vi "Host - Launch Target VIs (SubVI).vi"(8 "error in":errorcluster, 11 "IP":string[](array[string])) -> (0 "error out":errorcluster, 1 "VI Ref":refnum<vi>[](array[refnum]), 2 "Channel Data":cluster{"AI":T5, "DI":T2, "DO":T2, "Async":T9}[](array[cluster]) {"AI"."Interface Data"."Timing"."sample mode" items=["Finite Samples"=10178, "Continuous Samples"=10123, "Hardware Timed Single Point"=12522]; "Async"."Interface Data"."Data"."Minor Frame Count" min=5 max=8 step=1}, 3 "DO":T2[](array[typedef]), 7 "DI":T2[](array[typedef]))   [LabVIEW 2021]
uses:
  Async Serial/Controls/Async Message Info Cluster.ctl
  Async Serial/Controls/Async Frame Info Cluster.ctl
  Async Serial/Controls/Async Serial Configuration Cluster.ctl
  Async Interface Data Cluster.ctl
  Async JSON Cluster.ctl
  Digital Output/SubVIs/Digital Dynamic Cluster.ctl
  Digital Output/Controls/DIO Interface Data.ctl
  Digital Output/Controls/DIO Configuration cluster.ctl
  Analog Output/Controls/AO Timing Cluster.ctl
  Analog Output/Controls/AO Channel Configuration Cluster.ctl
  Analog Output/Controls/AO Interface Data Cluster.ctl
  Analog Output/Controls/AO JSON Data Cluster.ctl
  Async Serial/Controls/Async Sensor Type.ctl
panel:
  in  "Sensor Type":T1=enum."INS"
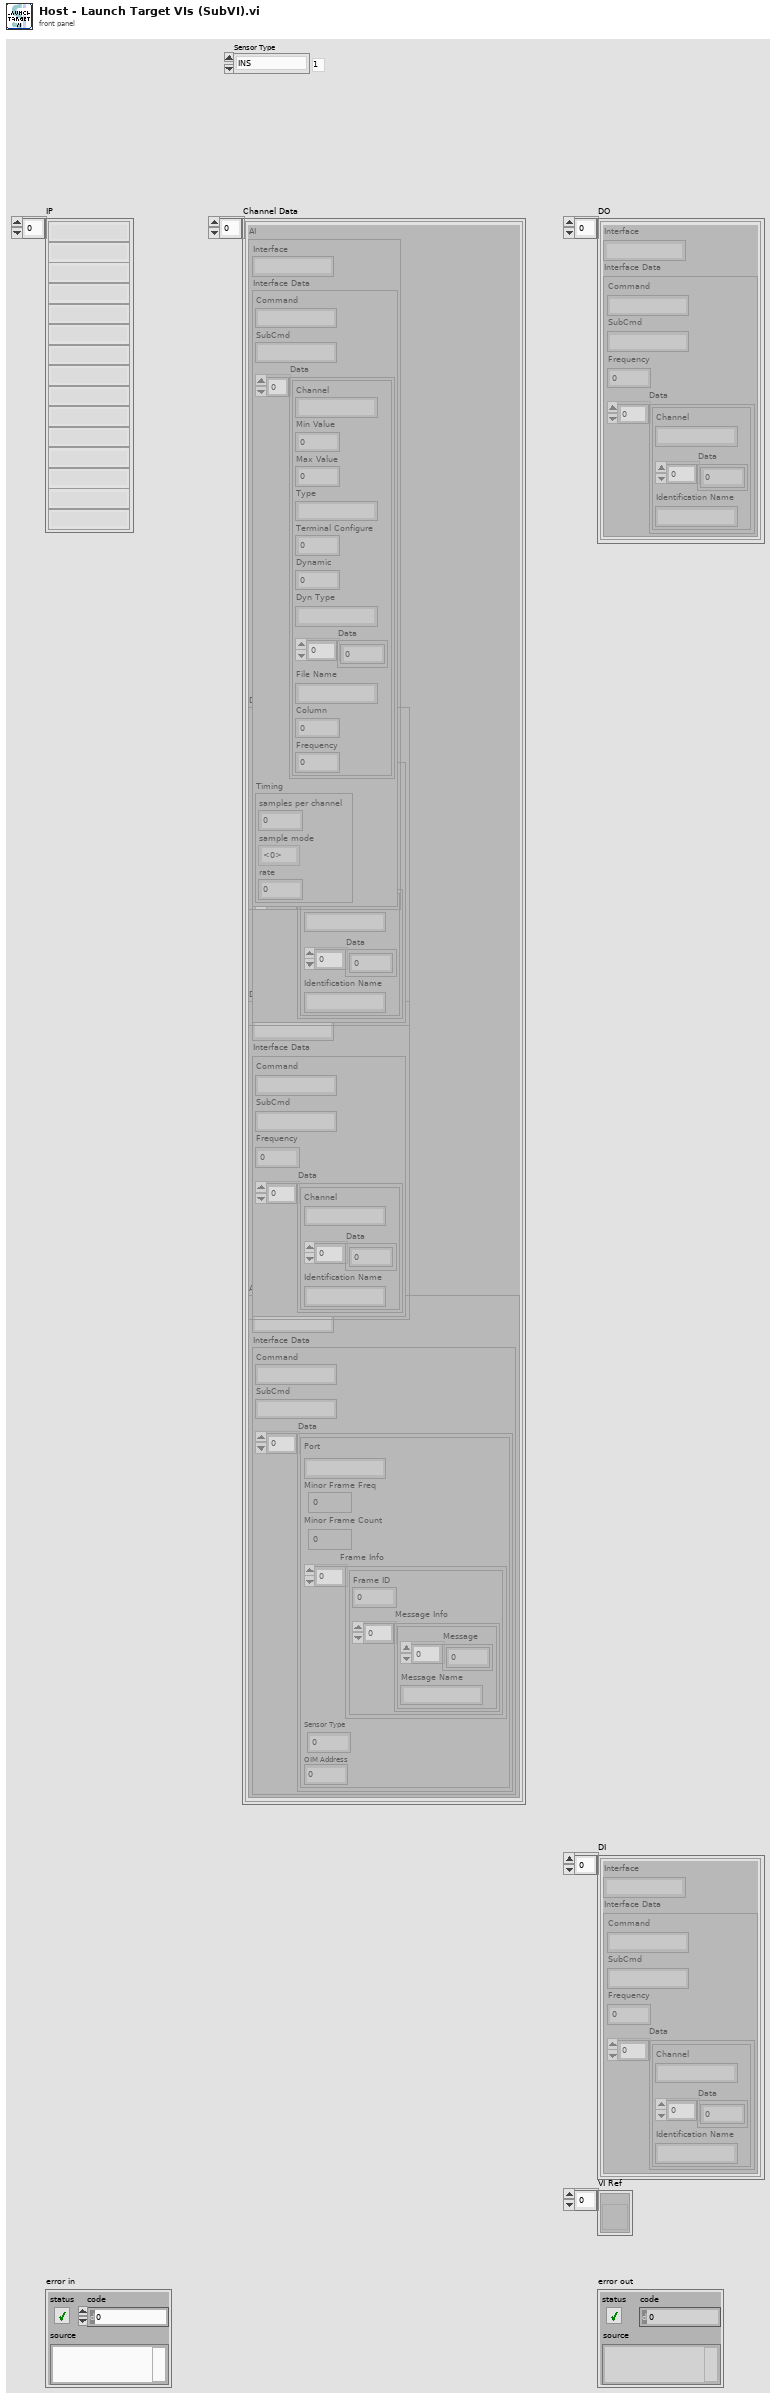
[diagram p1: front panel]
types:
  T1 = typedef "Async Sensor Type.ctl" = enum16{"Camera", "INS", "Pri BMS", "Aux BMS", "Depth Sensor", "Altimeter", "OIM", "Thruster", "Acoustic Modem", "LED"}
  T2 = typedef "DIO Configuration cluster.ctl" = cluster{"Interface":string, "Interface Data":T3}
  T3 = typedef "DIO Interface Data.ctl" = cluster{"Command":string, "SubCmd":string, "Frequency":u16, "Data":T4[]}
  T4 = typedef "Digital Dynamic Cluster.ctl" = cluster{"Channel":string, "Data":u8[], "Identification Name":string}
  T5 = typedef "AO JSON Data Cluster.ctl" = cluster{"Interface":string, "Interface Data":T6}
  T6 = typedef "AO Interface Data Cluster.ctl" = cluster{"Command":string, "SubCmd":string, "Data":T7[], "Timing":T8}
  T7 = typedef "AO Channel Configuration Cluster.ctl" = cluster{"Channel":string, "Min Value":dbl, "Max Value":dbl, "Type":string, "Terminal Configure":u16, "Dynamic":u8, "Dyn Type":string, "Data":dbl[], "File Name":string, "Column":i32, "Frequency":dbl}
  T8 = typedef "AO Timing Cluster.ctl" = cluster{"samples per channel":i32, "sample mode":i32, "rate":dbl}
  T9 = typedef "Async JSON Cluster.ctl" = cluster{"Interface":string, "Interface Data":T10}
  T10 = typedef "Async Interface Data Cluster.ctl" = cluster{"Command":string, "SubCmd":string, "Data":T11[]}
  T11 = typedef "Async Serial Configuration Cluster.ctl" = cluster{"Port":string, "Minor Frame Freq":u16, "Minor Frame Count":u16, "Frame Info":T12[], "Sensor Type":u16, "OIM Address":u16}
  T12 = typedef "Async Frame Info Cluster.ctl" = cluster{"Frame ID":u16, "Message Info":T13[]}
  T13 = typedef "Async Message Info Cluster.ctl" = cluster{"Message":u8[], "Message Name":string}
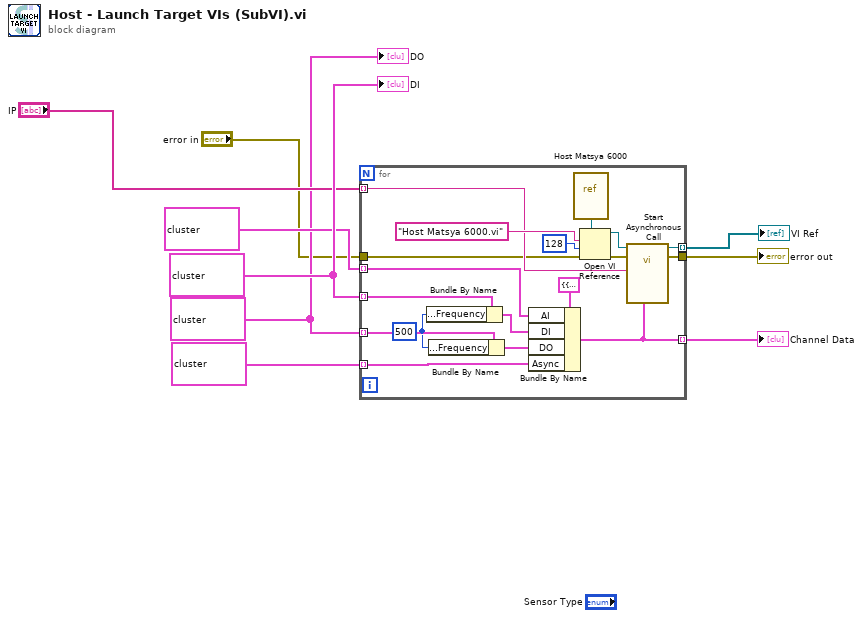
[diagram p0: block diagram]
diagram:
  w9 = T2[] [{"Interface"="DIO", "Interface Data"={"Command"="Configure", "SubCmd"="DI", "Frequency"=500, "Data"=[{"Channel"="Mod3/port0/line0", "Data"=[0], "Identification Name"=""}, {"Channel"="Mod3/port0/line1", "Data"=[0], "Identification Name"=""}, {"Channel"="Mod3/port0/line2", "Data"=[0], "Identification Name"=""}, {"Channel"="Mod3/port0/line3", "Data"=[0], "Identification Name"=""}, {"Channel"="Mod3/port0/line4", "Data"=[0], "Identification Name"=""}, {"Channel"="Mod3/port0/line5", "Data"=[0], "Identification Name"=""}, {"Channel"="Mod3/port0/line6", "Data"=[0], "Identification Name"=""}, {"Channel"="Mod3/port0/line7", "Data"=[0], "Identification Name"=""}, {"Channel"="Mod3/port0/line8", "Data"=[0], "Identification Name"=""}, {"Channel"="Mod3/port0/line9", "Data"=[0], "Identification Name"=""}, {"Channel"="Mod3/port0/line10", "Data"=[0], "Identification Name"=""}, {"Channel"="Mod3/port0/line11", "Data"=[0], "Identification Name"=""}, {"Channel"="Mod3/port0/line12", "Data"=[0], "Identification Name"=""}, {"Channel"="Mod3/port0/line13", "Data"=[0], "Identification Name"=""}, {"Channel"="Mod3/port0/line14", "Data"=[0], "Identification Name"=""}, {"Channel"="Mod3/port0/line15", "Data"=[0], "Identification Name"=""}, {"Channel"="Mod3/port0/line16", "Data"=[0], "Identification Name"=""}, {"Channel"="Mod3/port0/line17", "Data"=[0], "Identification Name"=""}, {"Channel"="Mod3/port0/line18", "Data"=[0], "Identification Name"=""}, {"Channel"="Mod3/port0/line19", "Data"=[0], "Identification Name"=""}, {"Channel"="Mod3/port0/line20", "Data"=[0], "Identification Name"=""}, {"Channel"="Mod3/port0/line21", "Data"=[0], "Identification Name"=""}, {"Channel"="Mod3/port0/line22", "Data"=[0], "Identification Name"=""}, {"Channel"="Mod3/port0/line23", "Data"=[0], "Identification Name"=""}, {"Channel"="Mod3/port0/line24", "Data"=[0], "Identification Name"=""}, {"Channel"="Mod3/port0/line25", "Data"=[0], "Identification Name"=""}, {"Channel"="Mod3/port0/line26", "Data"=[0], "Identification Name"=""}, {"Channel"="Mod3/port0/line27", "Data"=[0], "Identification Name"=""}, {"Channel"="Mod3/port0/line28", "Data"=[0], "Identification Name"=""}, {"Channel"="Mod3/port0/line29", "Data"=[0], "Identification Name"=""}, {"Channel"="Mod3/port0/line30", "Data"=[0], "Identification Name"=""}, {"Channel"="Mod3/port0/line31", "Data"=[0], "Identification Name"=""}, {"Channel"="Mod4/port0/line0", "Data"=[0], "Identification Name"=""}, {"Channel"="Mod4/port0/line1", "Data"=[0], "Identification Name"=""}, {"Channel"="Mod4/port0/line2", "Data"=[0], "Identification Name"=""}, {"Channel"="Mod4/port0/line3", "Data"=[0], "Identification Name"=""}, {"Channel"="Mod4/port0/line4", "Data"=[0], "Identification Name"=""}, {"Channel"="Mod4/port0/line5", "Data"=[0], "Identification Name"=""}, {"Channel"="Mod4/port0/line6", "Data"=[0], "Identification Name"=""}, {"Channel"="Mod4/port0/line7", "Data"=[0], "Identification Name"=""}, {"Channel"="Mod4/port0/line8", "Data"=[0], "Identification Name"=""}, {"Channel"="Mod4/port0/line9", "Data"=[0], "Identification Name"=""}, {"Channel"="Mod4/port0/line10", "Data"=[0], "Identification Name"=""}, {"Channel"="Mod4/port0/line11", "Data"=[0], "Identification Name"=""}, {"Channel"="Mod4/port0/line12", "Data"=[0], "Identification Name"=""}, {"Channel"="Mod4/port0/line13", "Data"=[0], "Identification Name"=""}, {"Channel"="Mod4/port0/line14", "Data"=[0], "Identification Name"=""}, {"Channel"="Mod4/port0/line15", "Data"=[0], "Identification Name"=""}, {"Channel"="Mod4/port0/line16", "Data"=[0], "Identification Name"=""}, {"Channel"="Mod4/port0/line17", "Data"=[0], "Identification Name"=""}, {"Channel"="Mod4/port0/line18", "Data"=[0], "Identification Name"=""}, {"Channel"="Mod4/port0/line19", "Data"=[0], "Identification Name"=""}, {"Channel"="Mod4/port0/line20", "Data"=[0], "Identification Name"=""}, {"Channel"="Mod4/port0/line21", "Data"=[0], "Identification Name"=""}, {"Channel"="Mod4/port0/line22", "Data"=[0], "Identification Name"=""}, {"Channel"="Mod4/port0/line23", "Data"=[0], "Identification Name"=""}, {"Channel"="Mod4/port0/line24", "Data"=[0], "Identification Name"=""}, {"Channel"="Mod4/port0/line25", "Data"=[0], "Identification Name"=""}, {"Channel"="Mod4/port0/line26", "Data"=[0], "Identification Name"=""}, {"Channel"="Mod4/port0/line27", "Data"=[0], "Identification Name"=""}, {"Channel"="Mod4/port0/line28", "Data"=[0], "Identification Name"=""}, {"Channel"="Mod4/port0/line29", "Data"=[0], "Identification Name"=""}, {"Channel"="Mod4/port0/line30", "Data"=[0], "Identification Name"=""}, {"Channel"="Mod4/port0/line31", "Data"=[0], "Identification Name"=""}]}}, {"Interface"="DIO", "Interface Data"={"Command"="", "SubCmd"="DI", "Frequency"=500, "Data"=[]}}, {"Interface"="DIO", "Interface Data"={"Command"="Configure", "SubCmd"="DI", "Frequency"=500, "Data"=[{"Channel"="Mod3/port0/line0", "Data"=[0], "Identification Name"=""}, {"Channel"="Mod3/port0/line1", "Data"=[0], "Identification Name"=""}, {"Channel"="Mod3/port0/line2", "Data"=[0], "Identification Name"=""}, {"Channel"="Mod3/port0/line3", "Data"=[0], "Identification Name"=""}, {"Channel"="Mod3/port0/line4", "Data"=[0], "Identification Name"=""}, {"Channel"="Mod3/port0/line5", "Data"=[0], "Identification Name"=""}, {"Channel"="Mod3/port0/line6", "Data"=[0], "Identification Name"=""}, {"Channel"="Mod3/port0/line7", "Data"=[0], "Identification Name"=""}, {"Channel"="Mod3/port0/line8", "Data"=[0], "Identification Name"=""}, {"Channel"="Mod3/port0/line9", "Data"=[0], "Identification Name"=""}, {"Channel"="Mod3/port0/line10", "Data"=[0], "Identification Name"=""}, {"Channel"="Mod3/port0/line11", "Data"=[0], "Identification Name"=""}, {"Channel"="Mod3/port0/line12", "Data"=[0], "Identification Name"=""}, {"Channel"="Mod3/port0/line13", "Data"=[0], "Identification Name"=""}, {"Channel"="Mod3/port0/line14", "Data"=[0], "Identification Name"=""}, {"Channel"="Mod3/port0/line15", "Data"=[0], "Identification Name"=""}, {"Channel"="Mod3/port0/line16", "Data"=[0], "Identification Name"=""}, {"Channel"="Mod3/port0/line17", "Data"=[0], "Identification Name"=""}, {"Channel"="Mod3/port0/line18", "Data"=[0], "Identification Name"=""}, {"Channel"="Mod3/port0/line19", "Data"=[0], "Identification Name"=""}, {"Channel"="Mod3/port0/line20", "Data"=[0], "Identification Name"=""}, {"Channel"="Mod3/port0/line21", "Data"=[0], "Identification Name"=""}, {"Channel"="Mod3/port0/line22", "Data"=[0], "Identification Name"=""}, {"Channel"="Mod3/port0/line23", "Data"=[0], "Identification Name"=""}, {"Channel"="Mod3/port0/line24", "Data"=[0], "Identification Name"=""}, {"Channel"="Mod3/port0/line25", "Data"=[0], "Identification Name"=""}, {"Channel"="Mod3/port0/line26", "Data"=[0], "Identification Name"=""}, {"Channel"="Mod3/port0/line27", "Data"=[0], "Identification Name"=""}, {"Channel"="Mod3/port0/line28", "Data"=[0], "Identification Name"=""}, {"Channel"="Mod3/port0/line29", "Data"=[0], "Identification Name"=""}, {"Channel"="Mod3/port0/line30", "Data"=[0], "Identification Name"=""}, {"Channel"="Mod3/port0/line31", "Data"=[0], "Identification Name"=""}, {"Channel"="Mod4/port0/line0", "Data"=[0], "Identification Name"=""}, {"Channel"="Mod4/port0/line1", "Data"=[0], "Identification Name"=""}, {"Channel"="Mod4/port0/line2", "Data"=[0], "Identification Name"=""}, {"Channel"="Mod4/port0/line3", "Data"=[0], "Identification Name"=""}, {"Channel"="Mod4/port0/line4", "Data"=[0], "Identification Name"=""}, {"Channel"="Mod4/port0/line5", "Data"=[0], "Identification Name"=""}, {"Channel"="Mod4/port0/line6", "Data"=[0], "Identification Name"=""}, {"Channel"="Mod4/port0/line7", "Data"=[0], "Identification Name"=""}, {"Channel"="Mod4/port0/line8", "Data"=[0], "Identification Name"=""}, {"Channel"="Mod4/port0/line9", "Data"=[0], "Identification Name"=""}, {"Channel"="Mod4/port0/line10", "Data"=[0], "Identification Name"=""}, {"Channel"="Mod4/port0/line11", "Data"=[0], "Identification Name"=""}, {"Channel"="Mod4/port0/line12", "Data"=[0], "Identification Name"=""}, {"Channel"="Mod4/port0/line13", "Data"=[0], "Identification Name"=""}, {"Channel"="Mod4/port0/line14", "Data"=[0], "Identification Name"=""}, {"Channel"="Mod4/port0/line15", "Data"=[0], "Identification Name"=""}, {"Channel"="Mod4/port0/line16", "Data"=[0], "Identification Name"=""}, {"Channel"="Mod4/port0/line17", "Data"=[0], "Identification Name"=""}, {"Channel"="Mod4/port0/line18", "Data"=[0], "Identification Name"=""}, {"Channel"="Mod4/port0/line19", "Data"=[0], "Identification Name"=""}, {"Channel"="Mod4/port0/line20", "Data"=[0], "Identification Name"=""}, {"Channel"="Mod4/port0/line21", "Data"=[0], "Identification Name"=""}, {"Channel"="Mod4/port0/line22", "Data"=[0], "Identification Name"=""}, {"Channel"="Mod4/port0/line23", "Data"=[0], "Identification Name"=""}, {"Channel"="Mod4/port0/line24", "Data"=[0], "Identification Name"=""}, {"Channel"="Mod4/port0/line25", "Data"=[0], "Identification Name"=""}, {"Channel"="Mod4/port0/line26", "Data"=[0], "Identification Name"=""}, {"Channel"="Mod4/port0/line27", "Data"=[0], "Identification Name"=""}, {"Channel"="Mod4/port0/line28", "Data"=[0], "Identification Name"=""}, {"Channel"="Mod4/port0/line29", "Data"=[0], "Identification Name"=""}, {"Channel"="Mod4/port0/line30", "Data"=[0], "Identification Name"=""}, {"Channel"="Mod4/port0/line31", "Data"=[0], "Identification Name"=""}]}}, {"Interface"="DIO", "Interface Data"={"Command"="Configure", "SubCmd"="DI", "Frequency"=500, "Data"=[]}}, {"Interface"="DIO", "Interface Data"={"Command"="Configure", "SubCmd"="DI", "Frequency"=500, "Data"=[]}}, {"Interface"="DIO", "Interface Data"={"Command"="Configure", "SubCmd"="DI", "Frequency"=500, "Data"=[]}}] ("DI 2")
  w2 = T2[] [{"Interface"="DIO", "Interface Data"={"Command"="Configure", "SubCmd"="DO", "Frequency"=500, "Data"=[{"Channel"="Mod1/port0/line0", "Data"=[0], "Identification Name"=""}, {"Channel"="Mod1/port0/line1", "Data"=[0], "Identification Name"=""}, {"Channel"="Mod1/port0/line2", "Data"=[0], "Identification Name"=""}, {"Channel"="Mod1/port0/line3", "Data"=[0], "Identification Name"=""}, {"Channel"="Mod1/port0/line4", "Data"=[0], "Identification Name"=""}, {"Channel"="Mod1/port0/line5", "Data"=[0], "Identification Name"=""}, {"Channel"="Mod1/port0/line6", "Data"=[0], "Identification Name"=""}, {"Channel"="Mod1/port0/line7", "Data"=[0], "Identification Name"=""}, {"Channel"="Mod1/port0/line8", "Data"=[0], "Identification Name"=""}, {"Channel"="Mod1/port0/line9", "Data"=[0], "Identification Name"=""}, {"Channel"="Mod1/port0/line10", "Data"=[0], "Identification Name"=""}, {"Channel"="Mod1/port0/line11", "Data"=[0], "Identification Name"=""}, {"Channel"="Mod1/port0/line12", "Data"=[0], "Identification Name"=""}, {"Channel"="Mod1/port0/line13", "Data"=[0], "Identification Name"=""}, {"Channel"="Mod1/port0/line14", "Data"=[0], "Identification Name"=""}, {"Channel"="Mod1/port0/line15", "Data"=[0], "Identification Name"=""}, {"Channel"="Mod1/port0/line16", "Data"=[0], "Identification Name"=""}, {"Channel"="Mod1/port0/line17", "Data"=[0], "Identification Name"=""}, {"Channel"="Mod1/port0/line18", "Data"=[0], "Identification Name"=""}, {"Channel"="Mod1/port0/line19", "Data"=[0], "Identification Name"=""}, {"Channel"="Mod1/port0/line20", "Data"=[0], "Identification Name"=""}, {"Channel"="Mod1/port0/line21", "Data"=[0], "Identification Name"=""}, {"Channel"="Mod1/port0/line22", "Data"=[0], "Identification Name"=""}, {"Channel"="Mod1/port0/line23", "Data"=[0], "Identification Name"=""}, {"Channel"="Mod1/port0/line24", "Data"=[0], "Identification Name"=""}, {"Channel"="Mod1/port0/line25", "Data"=[0], "Identification Name"=""}, {"Channel"="Mod1/port0/line26", "Data"=[0], "Identification Name"=""}, {"Channel"="Mod1/port0/line27", "Data"=[0], "Identification Name"=""}, {"Channel"="Mod1/port0/line28", "Data"=[0], "Identification Name"=""}, {"Channel"="Mod1/port0/line29", "Data"=[0], "Identification Name"=""}, {"Channel"="Mod1/port0/line30", "Data"=[0], "Identification Name"=""}, {"Channel"="Mod1/port0/line31", "Data"=[0], "Identification Name"=""}]}}, {"Interface"="DIO", "Interface Data"={"Command"="Configure", "SubCmd"="DO", "Frequency"=500, "Data"=[{"Channel"="Mod1/port0/line0", "Data"=[0], "Identification Name"=""}, {"Channel"="Mod1/port0/line1", "Data"=[0], "Identification Name"=""}, {"Channel"="Mod1/port0/line2", "Data"=[0], "Identification Name"=""}, {"Channel"="Mod1/port0/line3", "Data"=[0], "Identification Name"=""}, {"Channel"="Mod1/port0/line4", "Data"=[0], "Identification Name"=""}, {"Channel"="Mod1/port0/line5", "Data"=[0], "Identification Name"=""}, {"Channel"="Mod1/port0/line6", "Data"=[0], "Identification Name"=""}, {"Channel"="Mod1/port0/line7", "Data"=[0], "Identification Name"=""}, {"Channel"="Mod1/port0/line8", "Data"=[0], "Identification Name"=""}, {"Channel"="Mod1/port0/line9", "Data"=[0], "Identification Name"=""}, {"Channel"="Mod1/port0/line10", "Data"=[0], "Identification Name"=""}, {"Channel"="Mod1/port0/line11", "Data"=[0], "Identification Name"=""}, {"Channel"="Mod1/port0/line12", "Data"=[0], "Identification Name"=""}, {"Channel"="Mod1/port0/line13", "Data"=[0], "Identification Name"=""}, {"Channel"="Mod1/port0/line14", "Data"=[0], "Identification Name"=""}, {"Channel"="Mod1/port0/line15", "Data"=[0], "Identification Name"=""}, {"Channel"="Mod1/port0/line16", "Data"=[0], "Identification Name"=""}, {"Channel"="Mod1/port0/line17", "Data"=[0], "Identification Name"=""}, {"Channel"="Mod1/port0/line18", "Data"=[0], "Identification Name"=""}, {"Channel"="Mod1/port0/line19", "Data"=[0], "Identification Name"=""}, {"Channel"="Mod1/port0/line20", "Data"=[0], "Identification Name"=""}, {"Channel"="Mod1/port0/line21", "Data"=[0], "Identification Name"=""}, {"Channel"="Mod1/port0/line22", "Data"=[0], "Identification Name"=""}, {"Channel"="Mod1/port0/line23", "Data"=[0], "Identification Name"=""}, {"Channel"="Mod1/port0/line24", "Data"=[0], "Identification Name"=""}, {"Channel"="Mod1/port0/line25", "Data"=[0], "Identification Name"=""}, {"Channel"="Mod1/port0/line26", "Data"=[0], "Identification Name"=""}, {"Channel"="Mod1/port0/line27", "Data"=[0], "Identification Name"=""}, {"Channel"="Mod1/port0/line28", "Data"=[0], "Identification Name"=""}, {"Channel"="Mod1/port0/line29", "Data"=[0], "Identification Name"=""}, {"Channel"="Mod1/port0/line30", "Data"=[0], "Identification Name"=""}, {"Channel"="Mod1/port0/line31", "Data"=[0], "Identification Name"=""}, {"Channel"="Mod2/port0/line0", "Data"=[0], "Identification Name"=""}, {"Channel"="Mod2/port0/line1", "Data"=[0], "Identification Name"=""}, {"Channel"="Mod2/port0/line2", "Data"=[0], "Identification Name"=""}, {"Channel"="Mod2/port0/line3", "Data"=[0], "Identification Name"=""}, {"Channel"="Mod2/port0/line4", "Data"=[0], "Identification Name"=""}, {"Channel"="Mod2/port0/line5", "Data"=[0], "Identification Name"=""}, {"Channel"="Mod2/port0/line6", "Data"=[0], "Identification Name"=""}, {"Channel"="Mod2/port0/line7", "Data"=[0], "Identification Name"=""}, {"Channel"="Mod2/port0/line8", "Data"=[0], "Identification Name"=""}]}}, {"Interface"="DIO", "Interface Data"={"Command"="Configure", "SubCmd"="DO", "Frequency"=500, "Data"=[{"Channel"="Mod1/port0/line0", "Data"=[0], "Identification Name"=""}, {"Channel"="Mod1/port0/line1", "Data"=[0], "Identification Name"=""}, {"Channel"="Mod1/port0/line2", "Data"=[0], "Identification Name"=""}, {"Channel"="Mod1/port0/line3", "Data"=[0], "Identification Name"=""}, {"Channel"="Mod1/port0/line4", "Data"=[0], "Identification Name"=""}, {"Channel"="Mod1/port0/line5", "Data"=[0], "Identification Name"=""}, {"Channel"="Mod1/port0/line6", "Data"=[], "Identification Name"=""}, {"Channel"="Mod1/port0/line7", "Data"=[0], "Identification Name"=""}, {"Channel"="Mod1/port0/line8", "Data"=[0], "Identification Name"=""}, {"Channel"="Mod1/port0/line9", "Data"=[0], "Identification Name"=""}, {"Channel"="Mod1/port0/line10", "Data"=[0], "Identification Name"=""}, {"Channel"="Mod1/port0/line11", "Data"=[0], "Identification Name"=""}, {"Channel"="Mod1/port0/line12", "Data"=[0], "Identification Name"=""}, {"Channel"="Mod1/port0/line13", "Data"=[0], "Identification Name"=""}, {"Channel"="Mod1/port0/line14", "Data"=[0], "Identification Name"=""}, {"Channel"="Mod1/port0/line15", "Data"=[0], "Identification Name"=""}, {"Channel"="Mod1/port0/line16", "Data"=[0], "Identification Name"=""}, {"Channel"="Mod1/port0/line17", "Data"=[0], "Identification Name"=""}, {"Channel"="Mod1/port0/line18", "Data"=[0], "Identification Name"=""}, {"Channel"="Mod1/port0/line19", "Data"=[0], "Identification Name"=""}, {"Channel"="Mod1/port0/line20", "Data"=[0], "Identification Name"=""}, {"Channel"="Mod1/port0/line21", "Data"=[0], "Identification Name"=""}, {"Channel"="Mod1/port0/line22", "Data"=[0], "Identification Name"=""}, {"Channel"="Mod1/port0/line23", "Data"=[0], "Identification Name"=""}, {"Channel"="Mod1/port0/line24", "Data"=[0], "Identification Name"=""}, {"Channel"="Mod1/port0/line25", "Data"=[0], "Identification Name"=""}, {"Channel"="Mod1/port0/line26", "Data"=[0], "Identification Name"=""}, {"Channel"="Mod1/port0/line27", "Data"=[0], "Identification Name"=""}, {"Channel"="Mod1/port0/line28", "Data"=[0], "Identification Name"=""}, {"Channel"="Mod1/port0/line29", "Data"=[0], "Identification Name"=""}, {"Channel"="Mod1/port0/line30", "Data"=[0], "Identification Name"=""}, {"Channel"="Mod1/port0/line31", "Data"=[0], "Identification Name"=""}]}}, {"Interface"="DIO", "Interface Data"={"Command"="Configure", "SubCmd"="DO", "Frequency"=500, "Data"=[{"Channel"="Mod1/port0/line0", "Data"=[0], "Identification Name"=""}, {"Channel"="Mod1/port0/line1", "Data"=[0], "Identification Name"=""}, {"Channel"="Mod1/port0/line2", "Data"=[0], "Identification Name"=""}, {"Channel"="Mod1/port0/line3", "Data"=[0], "Identification Name"=""}, {"Channel"="Mod1/port0/line4", "Data"=[0], "Identification Name"=""}, {"Channel"="Mod1/port0/line5", "Data"=[0], "Identification Name"=""}, {"Channel"="Mod1/port0/line6", "Data"=[0], "Identification Name"=""}, {"Channel"="Mod1/port0/line7", "Data"=[0], "Identification Name"=""}, {"Channel"="Mod1/port0/line8", "Data"=[0], "Identification Name"=""}, {"Channel"="Mod1/port0/line9", "Data"=[0], "Identification Name"=""}, {"Channel"="Mod1/port0/line10", "Data"=[0], "Identification Name"=""}, {"Channel"="Mod1/port0/line11", "Data"=[0], "Identification Name"=""}, {"Channel"="Mod1/port0/line12", "Data"=[0], "Identification Name"=""}, {"Channel"="Mod1/port0/line13", "Data"=[0], "Identification Name"=""}, {"Channel"="Mod1/port0/line14", "Data"=[0], "Identification Name"=""}, {"Channel"="Mod1/port0/line15", "Data"=[0], "Identification Name"=""}, {"Channel"="Mod1/port0/line16", "Data"=[0], "Identification Name"=""}, {"Channel"="Mod1/port0/line17", "Data"=[0], "Identification Name"=""}, {"Channel"="Mod1/port0/line18", "Data"=[0], "Identification Name"=""}, {"Channel"="Mod1/port0/line19", "Data"=[0], "Identification Name"=""}, {"Channel"="Mod1/port0/line20", "Data"=[0], "Identification Name"=""}, {"Channel"="Mod1/port0/line21", "Data"=[0], "Identification Name"=""}, {"Channel"="Mod1/port0/line22", "Data"=[0], "Identification Name"=""}, {"Channel"="Mod1/port0/line23", "Data"=[0], "Identification Name"=""}, {"Channel"="Mod1/port0/line24", "Data"=[0], "Identification Name"=""}, {"Channel"="Mod1/port0/line25", "Data"=[0], "Identification Name"=""}, {"Channel"="Mod1/port0/line26", "Data"=[0], "Identification Name"=""}, {"Channel"="Mod1/port0/line27", "Data"=[0], "Identification Name"=""}, {"Channel"="Mod1/port0/line28", "Data"=[0], "Identification Name"=""}, {"Channel"="Mod1/port0/line29", "Data"=[0], "Identification Name"=""}, {"Channel"="Mod1/port0/line30", "Data"=[0], "Identification Name"=""}, {"Channel"="Mod1/port0/line31", "Data"=[0], "Identification Name"=""}]}}, {"Interface"="DIO", "Interface Data"={"Command"="Configure", "SubCmd"="DO", "Frequency"=500, "Data"=[{"Channel"="Mod1/port0/line0", "Data"=[0], "Identification Name"=""}, {"Channel"="Mod1/port0/line1", "Data"=[0], "Identification Name"=""}, {"Channel"="Mod1/port0/line2", "Data"=[0], "Identification Name"=""}, {"Channel"="Mod1/port0/line3", "Data"=[0], "Identification Name"=""}, {"Channel"="Mod1/port0/line4", "Data"=[0], "Identification Name"=""}, {"Channel"="Mod1/port0/line5", "Data"=[0], "Identification Name"=""}, {"Channel"="Mod1/port0/line6", "Data"=[0], "Identification Name"=""}, {"Channel"="Mod1/port0/line7", "Data"=[0], "Identification Name"=""}, {"Channel"="Mod1/port0/line8", "Data"=[0], "Identification Name"=""}, {"Channel"="Mod1/port0/line9", "Data"=[0], "Identification Name"=""}, {"Channel"="Mod1/port0/line10", "Data"=[0], "Identification Name"=""}, {"Channel"="Mod1/port0/line11", "Data"=[0], "Identification Name"=""}, {"Channel"="Mod1/port0/line12", "Data"=[0], "Identification Name"=""}, {"Channel"="Mod1/port0/line13", "Data"=[0], "Identification Name"=""}, {"Channel"="Mod1/port0/line14", "Data"=[0], "Identification Name"=""}, {"Channel"="Mod1/port0/line15", "Data"=[0], "Identification Name"=""}, {"Channel"="Mod1/port0/line16", "Data"=[0], "Identification Name"=""}, {"Channel"="Mod1/port0/line17", "Data"=[0], "Identification Name"=""}, {"Channel"="Mod1/port0/line18", "Data"=[0], "Identification Name"=""}, {"Channel"="Mod1/port0/line19", "Data"=[0], "Identification Name"=""}, {"Channel"="Mod1/port0/line20", "Data"=[0], "Identification Name"=""}, {"Channel"="Mod1/port0/line21", "Data"=[0], "Identification Name"=""}, {"Channel"="Mod1/port0/line22", "Data"=[0], "Identification Name"=""}, {"Channel"="Mod1/port0/line23", "Data"=[0], "Identification Name"=""}, {"Channel"="Mod1/port0/line24", "Data"=[0], "Identification Name"=""}, {"Channel"="Mod1/port0/line25", "Data"=[0], "Identification Name"=""}, {"Channel"="Mod1/port0/line26", "Data"=[0], "Identification Name"=""}, {"Channel"="Mod1/port0/line27", "Data"=[0], "Identification Name"=""}, {"Channel"="Mod1/port0/line28", "Data"=[0], "Identification Name"=""}, {"Channel"="Mod1/port0/line29", "Data"=[0], "Identification Name"=""}, {"Channel"="Mod1/port0/line30", "Data"=[0], "Identification Name"=""}, {"Channel"="Mod1/port0/line31", "Data"=[0], "Identification Name"=""}]}}, {"Interface"="DIO", "Interface Data"={"Command"="Configure", "SubCmd"="DO", "Frequency"=500, "Data"=[{"Channel"="Mod1/port0/line0", "Data"=[0], "Identification Name"=""}, {"Channel"="Mod1/port0/line1", "Data"=[0], "Identification Name"=""}, {"Channel"="Mod1/port0/line2", "Data"=[0], "Identification Name"=""}, {"Channel"="Mod1/port0/line3", "Data"=[0], "Identification Name"=""}, {"Channel"="Mod1/port0/line4", "Data"=[0], "Identification Name"=""}, {"Channel"="Mod1/port0/line5", "Data"=[0], "Identification Name"=""}, {"Channel"="Mod1/port0/line6", "Data"=[0], "Identification Name"=""}, {"Channel"="Mod1/port0/line7", "Data"=[0], "Identification Name"=""}, {"Channel"="Mod1/port0/line8", "Data"=[0], "Identification Name"=""}, {"Channel"="Mod1/port0/line9", "Data"=[0], "Identification Name"=""}, {"Channel"="Mod1/port0/line10", "Data"=[0], "Identification Name"=""}, {"Channel"="Mod1/port0/line11", "Data"=[0], "Identification Name"=""}, {"Channel"="Mod1/port0/line12", "Data"=[0], "Identification Name"=""}, {"Channel"="Mod1/port0/line13", "Data"=[0], "Identification Name"=""}, {"Channel"="Mod1/port0/line14", "Data"=[0], "Identification Name"=""}, {"Channel"="Mod1/port0/line15", "Data"=[0], "Identification Name"=""}, {"Channel"="Mod1/port0/line16", "Data"=[0], "Identification Name"=""}, {"Channel"="Mod1/port0/line17", "Data"=[0], "Identification Name"=""}, {"Channel"="Mod1/port0/line18", "Data"=[0], "Identification Name"=""}, {"Channel"="Mod1/port0/line19", "Data"=[0], "Identification Name"=""}, {"Channel"="Mod1/port0/line20", "Data"=[0], "Identification Name"=""}, {"Channel"="Mod1/port0/line21", "Data"=[0], "Identification Name"=""}, {"Channel"="Mod1/port0/line22", "Data"=[0], "Identification Name"=""}, {"Channel"="Mod1/port0/line23", "Data"=[0], "Identification Name"=""}, {"Channel"="Mod1/port0/line24", "Data"=[0], "Identification Name"=""}, {"Channel"="Mod1/port0/line25", "Data"=[0], "Identification Name"=""}, {"Channel"="Mod1/port0/line26", "Data"=[0], "Identification Name"=""}, {"Channel"="Mod1/port0/line27", "Data"=[0], "Identification Name"=""}, {"Channel"="Mod1/port0/line28", "Data"=[0], "Identification Name"=""}, {"Channel"="Mod1/port0/line29", "Data"=[0], "Identification Name"=""}, {"Channel"="Mod1/port0/line30", "Data"=[0], "Identification Name"=""}, {"Channel"="Mod1/port0/line31", "Data"=[0], "Identification Name"=""}, {"Channel"="Mod2/port0/line0", "Data"=[0], "Identification Name"=""}, {"Channel"="Mod2/port0/line1", "Data"=[0], "Identification Name"=""}, {"Channel"="Mod2/port0/line2", "Data"=[0], "Identification Name"=""}, {"Channel"="Mod2/port0/line3", "Data"=[0], "Identification Name"=""}, {"Channel"="Mod2/port0/line4", "Data"=[0], "Identification Name"=""}, {"Channel"="Mod2/port0/line5", "Data"=[0], "Identification Name"=""}, {"Channel"="Mod2/port0/line6", "Data"=[0], "Identification Name"=""}, {"Channel"="Mod2/port0/line7", "Data"=[0], "Identification Name"=""}, {"Channel"="Mod2/port0/line8", "Data"=[0], "Identification Name"=""}, {"Channel"="Mod2/port0/line9", "Data"=[0], "Identification Name"=""}, {"Channel"="Mod2/port0/line10", "Data"=[0], "Identification Name"=""}, {"Channel"="Mod2/port0/line11", "Data"=[0], "Identification Name"=""}, {"Channel"="Mod2/port0/line12", "Data"=[0], "Identification Name"=""}, {"Channel"="Mod2/port0/line13", "Data"=[0], "Identification Name"=""}, {"Channel"="Mod2/port0/line14", "Data"=[0], "Identification Name"=""}, {"Channel"="Mod2/port0/line15", "Data"=[0], "Identification Name"=""}, {"Channel"="Mod2/port0/line16", "Data"=[0], "Identification Name"=""}, {"Channel"="Mod2/port0/line17", "Data"=[0], "Identification Name"=""}, {"Channel"="Mod2/port0/line18", "Data"=[0], "Identification Name"=""}, {"Channel"="Mod2/port0/line19", "Data"=[0], "Identification Name"=""}, {"Channel"="Mod2/port0/line20", "Data"=[0], "Identification Name"=""}, {"Channel"="Mod2/port0/line21", "Data"=[0], "Identification Name"=""}, {"Channel"="Mod2/port0/line22", "Data"=[0], "Identification Name"=""}, {"Channel"="Mod2/port0/line23", "Data"=[0], "Identification Name"=""}, {"Channel"="Mod2/port0/line24", "Data"=[0], "Identification Name"=""}, {"Channel"="Mod2/port0/line25", "Data"=[0], "Identification Name"=""}, {"Channel"="Mod2/port0/line26", "Data"=[0], "Identification Name"=""}, {"Channel"="Mod2/port0/line27", "Data"=[0], "Identification Name"=""}, {"Channel"="Mod2/port0/line28", "Data"=[0], "Identification Name"=""}, {"Channel"="Mod2/port0/line29", "Data"=[0], "Identification Name"=""}, {"Channel"="Mod2/port0/line30", "Data"=[0], "Identification Name"=""}, {"Channel"="Mod2/port0/line31", "Data"=[0], "Identification Name"=""}]}}] ("DO")
  n1 = for {
    tunnel: "IP" -> [w23] mode=indexing
    tunnel: [w22] -> w5 mode=indexing
    tunnel: [w21] -> w7
    tunnel: w2 -> [w16] mode=indexing
    tunnel: T9[] [{"Interface"="Async", "Interface Data"={"Command"="Configure", "SubCmd"="Async", "Data"=[]}}, {"Interface"="Async", "Interface Data"={"Command"="Configure", "SubCmd"="Async", "Data"=[{"Port"="com1", "Minor Frame Freq"=200, "Minor Frame Count"=1, "Frame Info"=[{"Frame ID"=1, "Message Info"=[{"Message"=[1], "Message Name"="m1"}]}], "Sensor Type"=1, "OIM Address"=0}, {"Port"="com2", "Minor Frame Freq"=200, "Minor Frame Count"=1, "Frame Info"=[{"Frame ID"=1, "Message Info"=[{"Message"=[1], "Message Name"="LED"}]}], "Sensor Type"=9, "OIM Address"=0}, {"Port"="com10", "Minor Frame Freq"=200, "Minor Frame Count"=1, "Frame Info"=[{"Frame ID"=1, "Message Info"=[{"Message"=[1], "Message Name"="LED"}]}], "Sensor Type"=9, "OIM Address"=0}, {"Port"="com11", "Minor Frame Freq"=200, "Minor Frame Count"=1, "Frame Info"=[{"Frame ID"=1, "Message Info"=[{"Message"=[1], "Message Name"="LED"}]}], "Sensor Type"=9, "OIM Address"=0}]}}, {"Interface"="Async", "Interface Data"={"Command"="Configure", "SubCmd"="Async", "Data"=[]}}, {"Interface"="Async", "Interface Data"={"Command"="Configure", "SubCmd"="Async", "Data"=[{"Port"="com10", "Minor Frame Freq"=200, "Minor Frame Count"=5, "Frame Info"=[{"Frame ID"=1, "Message Info"=[{"Message"=[1], "Message Name"="m1"}]}], "Sensor Type"=7, "OIM Address"=0}, {"Port"="com11", "Minor Frame Freq"=200, "Minor Frame Count"=5, "Frame Info"=[{"Frame ID"=1, "Message Info"=[{"Message"=[1], "Message Name"="m1"}]}], "Sensor Type"=7, "OIM Address"=0}, {"Port"="com12", "Minor Frame Freq"=200, "Minor Frame Count"=5, "Frame Info"=[{"Frame ID"=1, "Message Info"=[{"Message"=[1], "Message Name"="m1"}]}], "Sensor Type"=7, "OIM Address"=0}, {"Port"="com13", "Minor Frame Freq"=200, "Minor Frame Count"=5, "Frame Info"=[{"Frame ID"=1, "Message Info"=[{"Message"=[1], "Message Name"="m1"}]}], "Sensor Type"=7, "OIM Address"=0}, {"Port"="com20", "Minor Frame Freq"=200, "Minor Frame Count"=5, "Frame Info"=[{"Frame ID"=1, "Message Info"=[{"Message"=[1], "Message Name"="m1"}]}], "Sensor Type"=6, "OIM Address"=4}, {"Port"="com21", "Minor Frame Freq"=200, "Minor Frame Count"=5, "Frame Info"=[{"Frame ID"=1, "Message Info"=[{"Message"=[1], "Message Name"="m1"}]}], "Sensor Type"=6, "OIM Address"=3}]}}, {"Interface"="Async", "Interface Data"={"Command"="Configure", "SubCmd"="Async", "Data"=[{"Port"="com10", "Minor Frame Freq"=200, "Minor Frame Count"=5, "Frame Info"=[{"Frame ID"=1, "Message Info"=[{"Message"=[1], "Message Name"="m1"}]}], "Sensor Type"=7, "OIM Address"=0}, {"Port"="com11", "Minor Frame Freq"=200, "Minor Frame Count"=5, "Frame Info"=[{"Frame ID"=1, "Message Info"=[{"Message"=[1], "Message Name"="m1"}]}], "Sensor Type"=7, "OIM Address"=0}, {"Port"="com12", "Minor Frame Freq"=200, "Minor Frame Count"=5, "Frame Info"=[{"Frame ID"=1, "Message Info"=[{"Message"=[1], "Message Name"="m1"}]}], "Sensor Type"=7, "OIM Address"=0}, {"Port"="com13", "Minor Frame Freq"=200, "Minor Frame Count"=5, "Frame Info"=[{"Frame ID"=1, "Message Info"=[{"Message"=[1], "Message Name"="m1"}]}], "Sensor Type"=7, "OIM Address"=0}]}}, {"Interface"="Async", "Interface Data"={"Command"="Configure", "SubCmd"="Async", "Data"=[{"Port"="com1", "Minor Frame Freq"=200, "Minor Frame Count"=8, "Frame Info"=[{"Frame ID"=1, "Message Info"=[{"Message"=[1, 0, 0, 0, 0, 0], "Message Name"="Camera cmd 1"}, {"Message"=[1, 0, 0, 0, 0, 0], "Message Name"="Camera cmd 2"}]}, {"Frame ID"=1, "Message Info"=[{"Message"=[1, 0, 0, 0, 0, 0], "Message Name"="Camera cmd 2"}, {"Message"=[1, 0, 0, 0, 0, 0], "Message Name"="Camera cmd 2"}]}], "Sensor Type"=0, "OIM Address"=0}]}}] ("Serial") -> [w15] mode=indexing
    tunnel: T5[] data[13084B] ("AI") -> [w18] mode=indexing
    tunnel: w9 -> [w17] mode=indexing
    tunnel: "error in" -> [w11]
    tunnel: [w10] -> w6 mode=indexing
    w12 = u16 500 ("Interface Data.Frequency")
    n2 = Bundle By Name(cluster=w17, "Interface Data.Frequency"=w12) -> (w14:T2)
    n3 = Bundle By Name(cluster=w16, "Interface Data.Frequency"=w12) -> (w13:T2)
    n4 = Bundle By Name(cluster=cluster{"AI":T5, "DI":T2, "DO":T2, "Async":T9} {"AI"={"Interface"="", "Interface Data"={"Command"="", "SubCmd"="", "Data"=[], "Timing"={"samples per channel"=0, "sample mode"=0, "rate"=0.0}}}, "DI"={"Interface"="", "Interface Data"={"Command"="", "SubCmd"="", "Frequency"=0, "Data"=[]}}, "DO"={"Interface"="", "Interface Data"={"Command"="", "SubCmd"="", "Frequency"=0, "Data"=[]}}, "Async"={"Interface"="", "Interface Data"={"Command"="", "SubCmd"="", "Data"=[]}}} ("Channel Data"), "AI"=w18, "DI"=w14, "DO"=w13, "Async"=w15) -> (w10:cluster{"AI":T5, "DI":T2, "DO":T2, "Async":T9})
    n5 = vi-ref "Host Matsya 6000.vi"() -> (w26:refnum<vi>)
    n6 = Open VI Reference(type specifier VI Refnum (for type only)=w26, vi path="Host Matsya 6000.vi", options=128, error in (no error)=w11) -> (vi reference=w27:refnum<vi>, error out=w20:errorcluster)  [unwired: 2 in]
    n7 = call-by-ref "Start Asynchronous Call"(reference=w27, error in=w20, "Channel Data"=w10, "address"=w23) -> (reference out=w22:refnum<vi>, error out=w21:errorcluster)  [unwired: 10 in]
  }
  "error out" <- w7
  "Channel Data" <- w6
  "VI Ref" <- w5
  "DI" <- w9
  "DO" <- w2
